vi "Actor Core.vi"(8 "error in":errorcluster, 11 "Browers in":refnum<class "Browers Controller.lvclass">) -> (0 "error out":errorcluster, 3 "Actor out":refnum<class "Actor.lvclass">)   [LabVIEW 2015, in "Browers Controller.lvclass"]
doc: "(<B>Filename</B>: Actor Framework.lvlib:Actor.lvclass:Actor Core.vi)\n\nReceives messages to the actor, reacts to them, and initiates any error handling that may shut the actor down.\n\nDescendant classes may override this VI to append parallel tasks for the actor to complete while it handles messages. Overrides use the Call Parent Method node."
uses:
  Browers Controller.lvclass
  <vilib>/ActorFramework/Actor/Actor.lvclass
  Menubar/Menu.lvclass
  Brower View/Type Definition/Brower Controls and VI Refnum.ctl
  Brower View/Brower View.lvclass
  Brower View/Brower View.lvclass/Brower View.ctl
  Browers Controller.lvclass/Browers Controller.ctl
  <vilib>/ActorFramework/Actor/Actor.lvclass/Actor.ctl
  <vilib>/ActorFramework/Message Enqueuer/Message Enqueuer.lvclass/Message Enqueuer.ctl
  <vilib>/ActorFramework/Stop Msg/Stop Msg.lvclass/Stop Msg.ctl
  <vilib>/ActorFramework/Message Enqueuer/Init from Existing Queue.vi
  <vilib>/ActorFramework/Message Enqueuer/Enqueue Critical.vi
  <vilib>/ActorFramework/Message Priority Queue/Priority Enqueue.vi
  <vilib>/ActorFramework/Message Enqueuer/Message Enqueuer.lvclass
  <vilib>/ActorFramework/Stop Msg/Stop Msg.lvclass
  MyTreeAPI/MyTreeAPI.lvclass
panel:
  in  "stop":bool
  in  "Brower":string(tree)
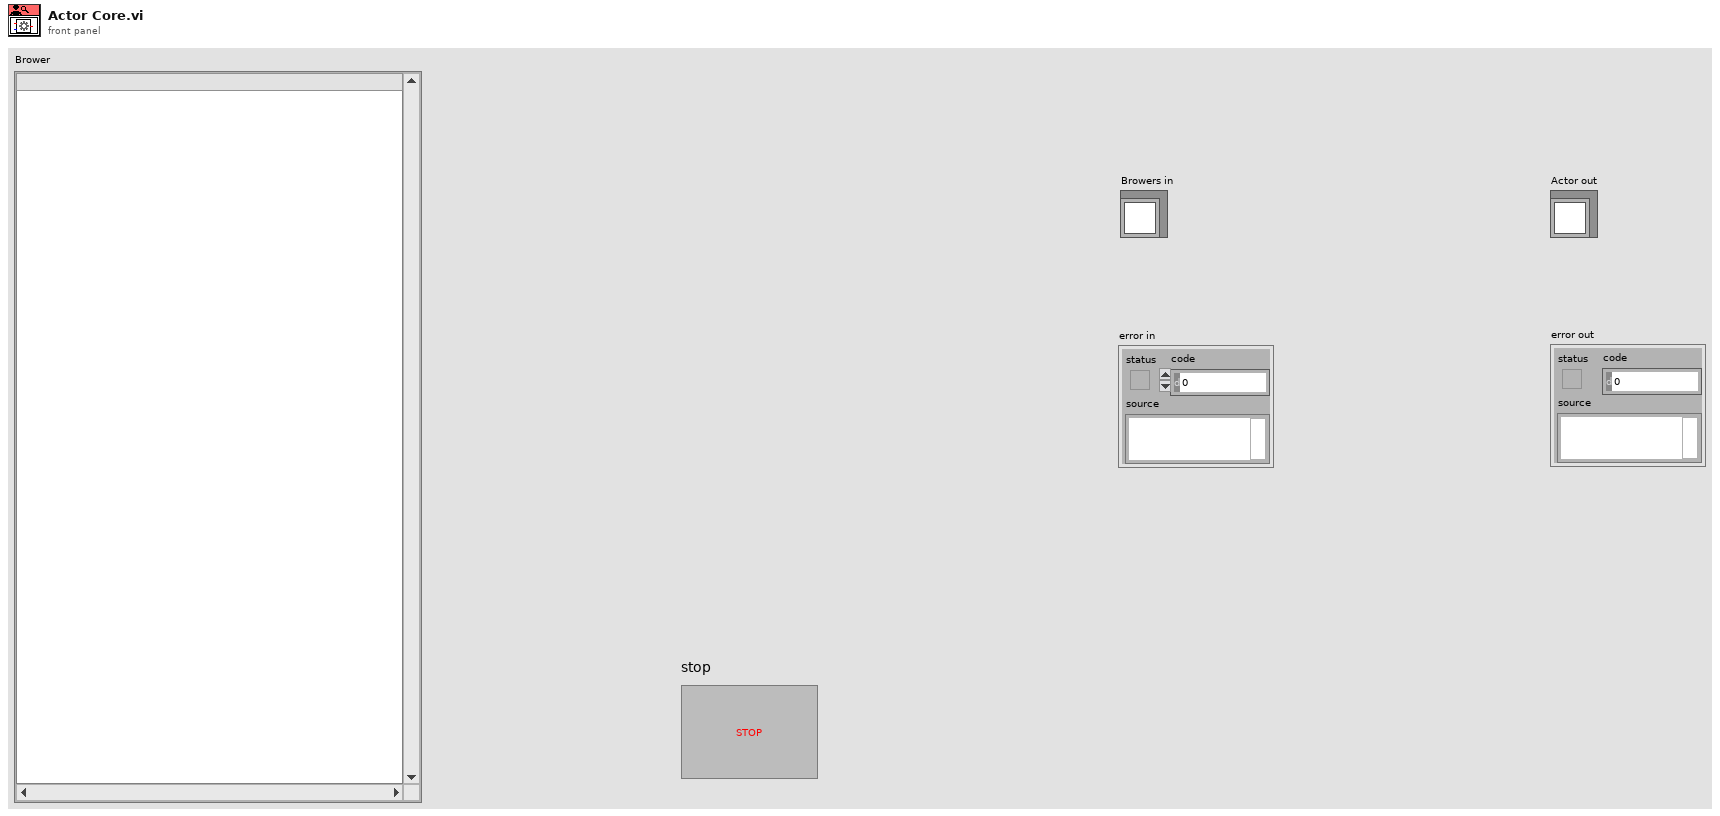
[diagram p1: front panel]
types:
  T1 = typedef "Brower View.lvclass/Brower Controls and VI Refnum.ctl" = cluster{"Brower":refnum<vi>, "This VI":refnum<vi>}
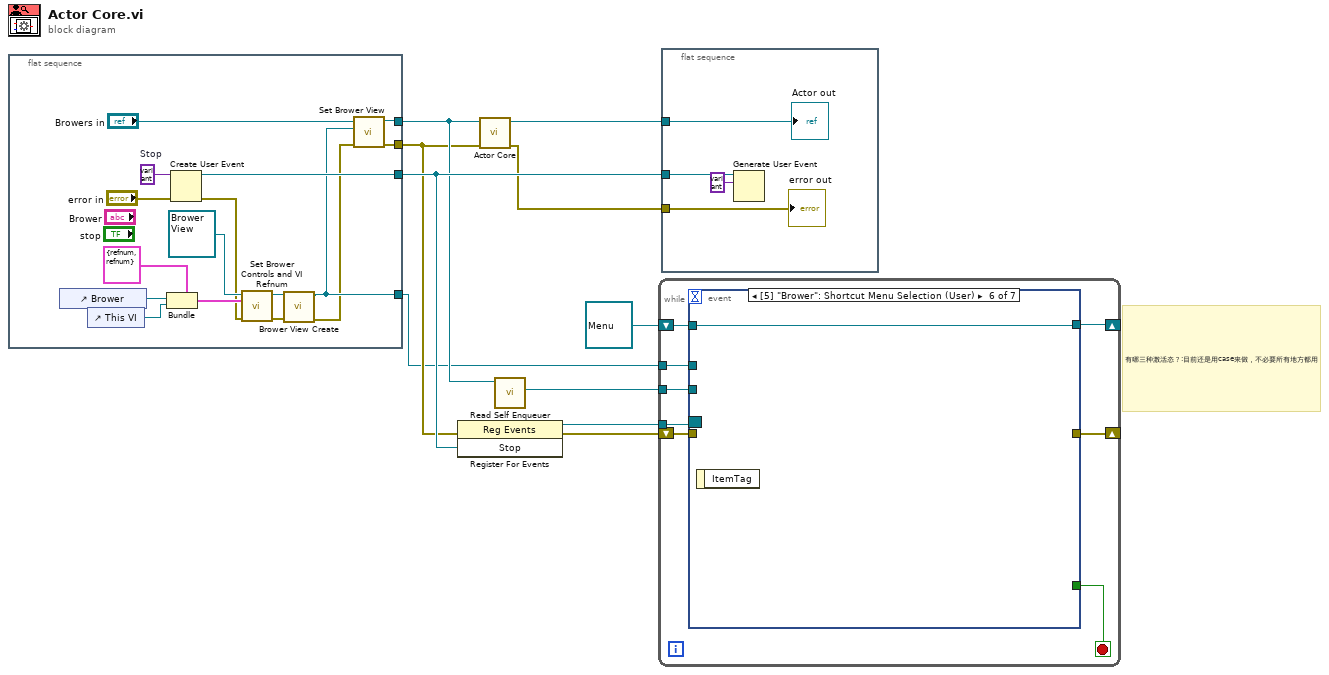
[diagram p0: block diagram]
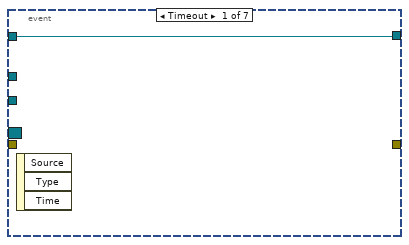
[diagram p2: hidden frame]
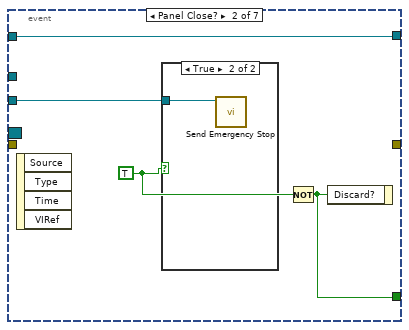
[diagram p3: hidden frame]
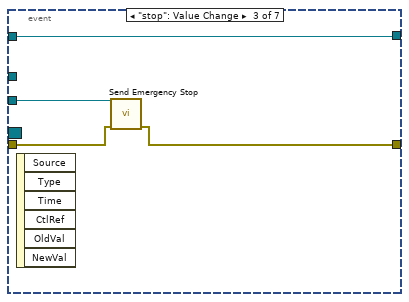
[diagram p5: hidden frame]
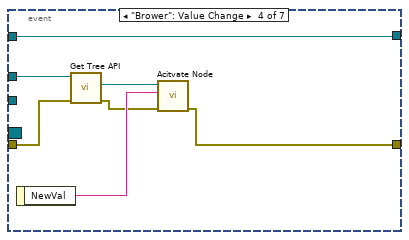
[diagram p6: hidden frame]
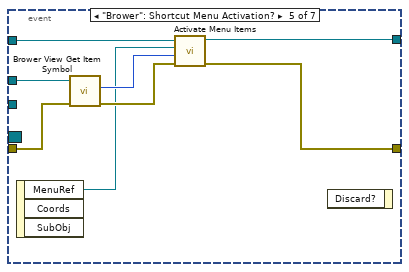
[diagram p7: hidden frame]
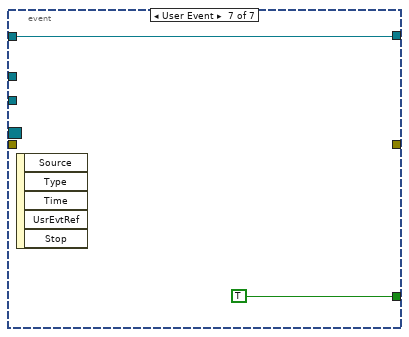
[diagram p8: hidden frame]
diagram:
  # "有哪三种激活态？:目前还是用case来做，不必要所有地方都用"
  n1 = flat-sequence {
    tunnel: [w25] -> w7
    tunnel: [w15] -> w4
    tunnel: [w17] -> w6
    tunnel: [w12] -> w2
    frame #0 {
      w26 = variant  # Stop
      n2 = control-ref of="Brower"() -> (w21:refnum<vi>)
      n3 = control-ref of="This VI"() -> (w22:refnum<vi>)
      n4 = Bundle(cluster=T1 {"Brower"=refnum, "This VI"=refnum}, "Brower"=w21, "This VI"=w22) -> (w19:T1)
      n5 = Create User Event(user event datatype=w26, error in="error in") -> (user event=w25:refnum<user-event>, error out=w16:errorcluster)
      n6 = call "Set Brower Controls and VI Refnum.vi"("error in (no error)"=w16, "Brower Controls and VI Refnum"=w19, "Brower View in"=refnum<class "Brower View.lvclass"> refnum) -> ("error out"=w13:errorcluster, "Brower View out"=w14:refnum<class "Brower View.lvclass">)  [unwired: 7 in]
      n7 = call "Brower View Create.vi"("error in (no error)"=w13, "Brower View in"=w14) -> ("error out"=w11:errorcluster, "Brower View out"=w12:refnum<class "Brower View.lvclass">)  [unwired: 8 in]
      n8 = call "Set Brower View .vi"("error in (no error)"=w11, "Brower View.lvclass"=w12, "Browers in"="Browers in") -> ("error out"=w15:errorcluster, "Browers out"=w17:refnum<class "Browers Controller.lvclass">)  [unwired: 7 in]
    }
  }
  n9 = register-events(error in=w4, w7) -> (reference out=w8:refnum<event-registration>, error out=w9:errorcluster)  [unwired: 1 in]
  n10 = call-parent "Actor Core.vi"("error in"=w4, "Actor in"=w6) -> ("error out"=w3:errorcluster, "Actor out"=w5:refnum<class "Actor.lvclass">)  [unwired: 8 in]
  n11 = call <vilib>:"Read Self Enqueuer.vi"("Actor"=w6) -> ("Self Enqueuer"=w10:refnum<class "Message Enqueuer.lvclass">)  [unwired: 10 in]
  n12 = while {
    tunnel: w8 -> [w34]
    tunnel: w10 -> [w33]
    tunnel: w2 -> [w30]
    shift-right: [w28] -> _
    shift-left: refnum<class "Menu.lvclass"> refnum ("Menu.lvclass") -> [w29]
    shift-right: [w27] -> _
    shift-left: w9 -> [w31]
    stop <- w32 stop-if-true
    n13 = event shown="[5] \"Brower\": Shortcut Menu Selection (User)" {
      selector: w34 -> [_ _ _ _ _ _ _]
      dyn-events: _ -> [_ _ _ _ _ _ _]
      timeout: _ -> [_ _ _ _ _ _ _]
      tunnel: w33 -> [_ w39 w44 _ _ _ _]
      tunnel: [_ w37 _ _ _ _ TRUE] -> w32
      tunnel: w31 -> [_ _ w43 w49 w58 _ _]
      tunnel: w30 -> [_ _ _ w50 w59 _ _]
      tunnel: w29 -> [w35 w36 w42 w51 w57 w60 w61]
      tunnel: [w35 w36 w42 w51 w54 w60 w61] -> w28
      tunnel: [_ _ w41 w45 w53 _ _] -> w27
      event Timeout {
        n14 = event-data() -> ()  [unwired: 1 in, 3 out]
      }
      event Panel Close? {
        w38 = TRUE
        n15 = event-data() -> ()  [unwired: 1 in, 4 out]
        n16 = case shown="True" w38 {
          tunnel: w39 -> [_ w40]
          frame False {
          }
          frame True {
            n17 = call <vilib>:"Send Emergency Stop.vi"("Message Enqueuer"=w40) -> ()  [unwired: 10 in, 1 out]
          }
        }
        n18 = Not(x=w38) -> (.not. x?=w37:bool)
        n19 = event-data("Discard?"=w37) -> ()  [unwired: 1 in, 1 out]
      }
      event "stop": Value Change {
        n20 = event-data() -> ()  [unwired: 1 in, 6 out]
        n21 = call <vilib>:"Send Emergency Stop.vi"("error in (no error)"=w43, "Message Enqueuer"=w44) -> ("error out"=w41:errorcluster)  [unwired: 9 in]
      }
      event "Brower": Value Change {
        n22 = event-data() -> ("NewVal"=w47:string)  [unwired: 1 in]
        n23 = call "Get Tree API.vi"("error in (no error)"=w49, "Brower View in"=w50) -> ("error out"=w46:errorcluster, "myTree.lvclass"=w48:refnum<class "MyTreeAPI.lvclass">)  [unwired: 7 in, 1 out]
        n24 = call "Acitvate Node.vi"("error in (no error)"=w46, "Active Node(\"\")"=w47, "TREE in"=w48) -> ("error out"=w45:errorcluster)  [unwired: 7 in, 1 out]
      }
      event "Brower": Shortcut Menu Activation? {
        n25 = event-data() -> ("MenuRef"=w52:refnum<k9>)  [unwired: 1 in, 2 out]
        n26 = call "Brower View Get Item Symbol.vi"("error in (no error)"=w58, "Brower View in"=w59) -> ("error out"=w56:errorcluster, "Symbol"=w55:i32)  [unwired: 7 in, 1 out]
        n27 = call-dynamic "Activate Menu Items.vi"("error in (no error)"=w56, "State(0)"=w55, "MenuRefnum"=w52, "Menu in"=w57) -> ("error out"=w53:errorcluster, "Menu out"=w54:refnum<class "Menu.lvclass">)  [unwired: 6 in]
        n28 = event-data() -> ()  [unwired: 2 in, 1 out]
      }
      event "Brower": Shortcut Menu Selection (User) {
        n29 = event-data() -> ()  [unwired: 1 in, 1 out]
      }
      event User Event {
        n30 = event-data() -> ()  [unwired: 1 in, 5 out]
      }
    }
  }
  n31 = flat-sequence {
    tunnel: w7 -> [w66]
    tunnel: w5 -> [w64]
    tunnel: w3 -> [w63]
    frame #0 {
      n32 = Generate User Event(user event=w66, event data cluster=variant ("event data")) -> ()  [unwired: 2 in, 2 out]
      "Actor out" <- w64
      "error out" <- w63
    }
  }
